vi "simple rig temperatures sim.vi"() -> (0 "Rig Temperatures":T1)   [LabVIEW 2018]
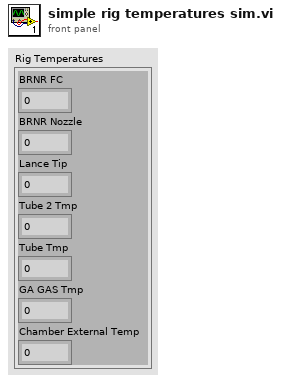
[diagram p1: front panel]
types:
  T1 = cluster{"BRNR FC":dbl, "BRNR Nozzle":dbl, "Lance Tip":dbl, "Tube 2 Tmp":dbl, "Tube Tmp":dbl, "GA GAS Tmp":dbl, "Chamber External Temp":dbl}
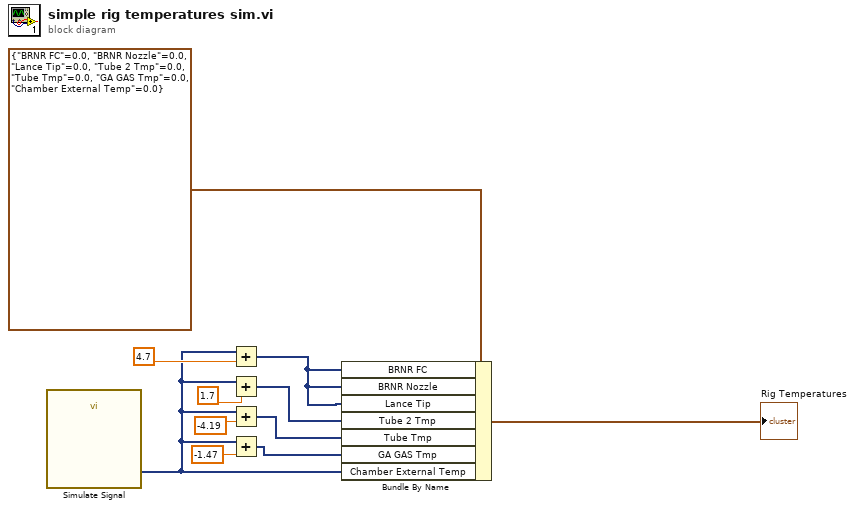
[diagram p0: block diagram]
diagram:
  n1 = call "Simulate Signal"() -> ("Rig Temperatures"=w2:dynamicdata)  [unwired: 14 in, 1 out]
  n2 = Add(x=w2, y=4.7) -> (x+y=w10:dynamicdata)
  n3 = Add(x=w2, y=1.7) -> (x+y=w8:dynamicdata)
  n4 = Add(x=w2, y=-4.19) -> (x+y=w6:dynamicdata)
  n5 = Add(x=w2, y=-1.47) -> (x+y=w4:dynamicdata)
  n6 = Bundle By Name(cluster=T1 {"BRNR FC"=0.0, "BRNR Nozzle"=0.0, "Lance Tip"=0.0, "Tube 2 Tmp"=0.0, "Tube Tmp"=0.0, "GA GAS Tmp"=0.0, "Chamber External Temp"=0.0}, "BRNR FC"=w10, "BRNR Nozzle"=w10, "Lance Tip"=w10, "Tube 2 Tmp"=w8, "Tube Tmp"=w6, "GA GAS Tmp"=w4, "Chamber External Temp"=w2) -> (→"Rig Temperatures":T1)
